vi "Hall sensor read-modify.vi"() -> ()   [LabVIEW 2013]
uses:
  <vilib>/measure/mascope.llb/Amplitude and Levels N chan.vi
  <vilib>/measure/NI_MAPro.lvlib
panel:
  in  "STOP":bool
  out "Anti-\nClockwise":bool
  out "Break\nCondition":bool
  out "Clockwise":bool
  out "No \nMagnetic\n    Field":bool
  out "North \n  Pole":bool
  out "South \n  Pole":bool
  out "PWM being applied\n(~Strength of magnetic field)":dbl
  out "Voltage Output- Hall Sensor":dynamicdata(graph)
  # "Hall Sensor Control"
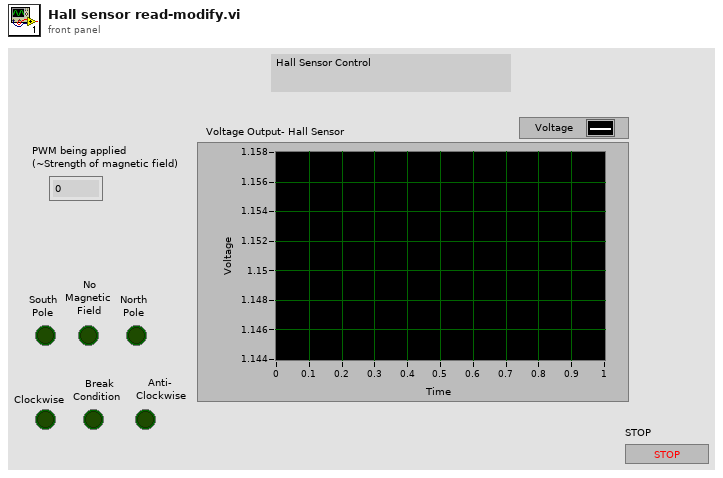
[diagram p1: front panel]
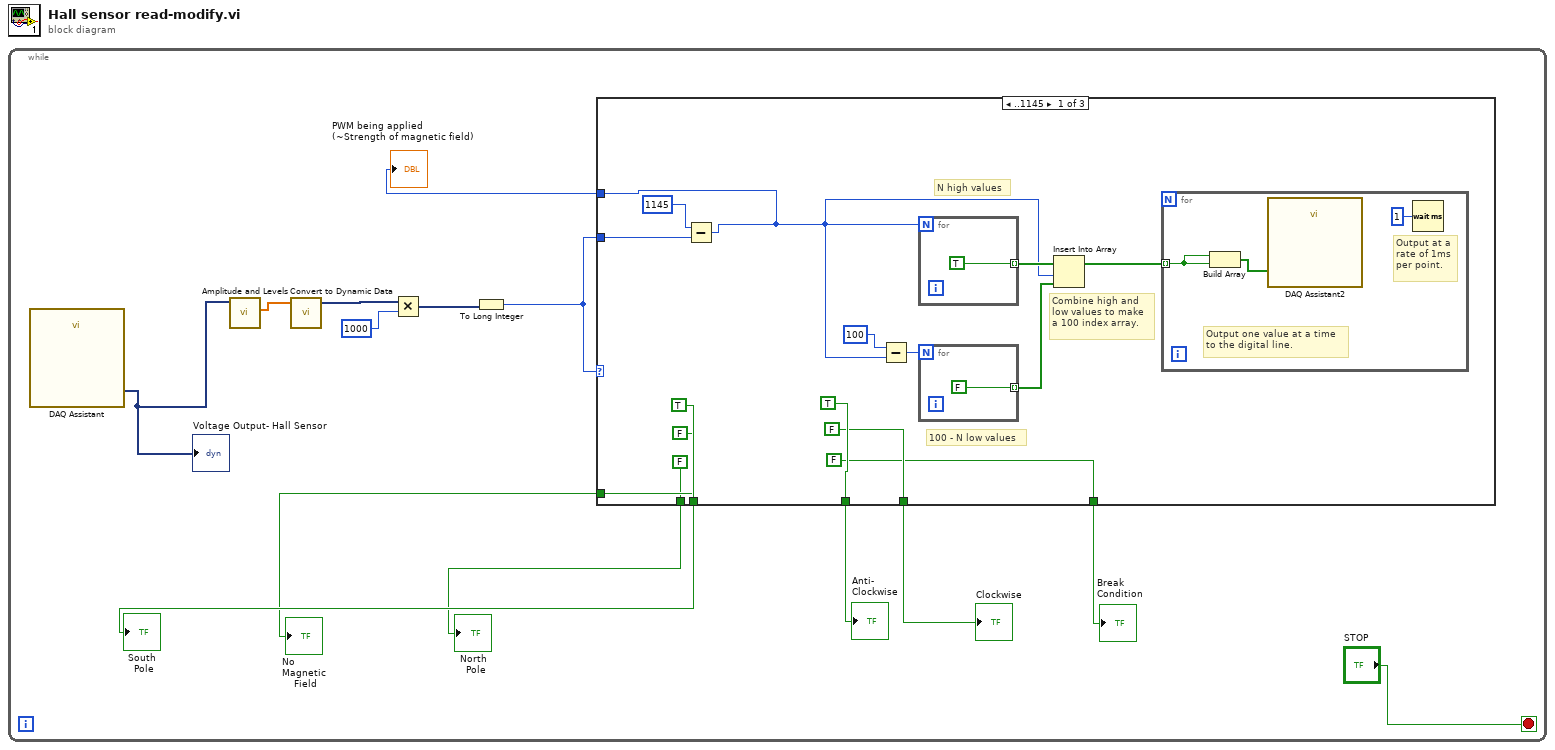
[diagram p0: block diagram]
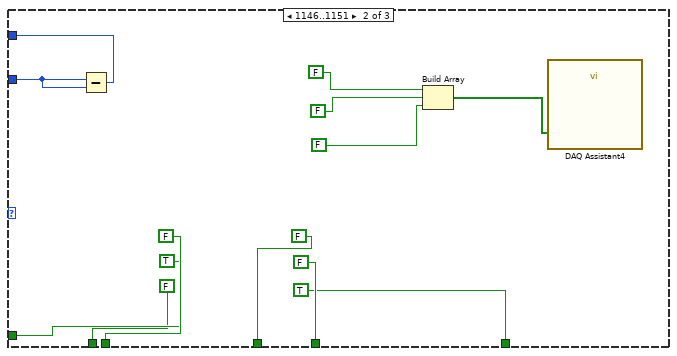
[diagram p2: hidden frame]
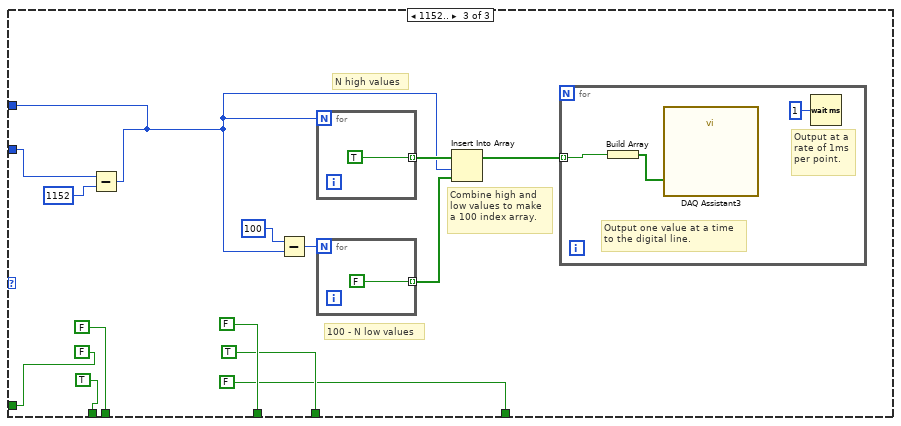
[diagram p3: hidden frame]
diagram:
  n1 = while {
    stop <- "STOP" stop-if-true
    n2 = call "DAQ Assistant"() -> ("data"=w14:dynamicdata)  [unwired: 17 in, 2 out]
    "Voltage Output- Hall Sensor" <- w14
    n3 = call-poly <vilib>:"Amplitude and Levels.vi"("signal(s) in"=w14) -> ("high state level"=w1:dbl[])  [unwired: 7 in, 3 out]
    n4 = call "Convert to Dynamic Data"("Array"=w1) -> ("Dynamic Data Type"=w12:dynamicdata)  [unwired: 3 in]
    n5 = Multiply(x=w12, y=1000) -> (x*y=w13:dynamicdata)
    n6 = To Long Integer(number=w13) -> (32bit integer=w10:i32)
    n7 = case shown="..1145" w10 {
      tunnel: w10 -> [w22 w41 w54]
      tunnel: [w21 w40 w52] -> w9
      tunnel: [TRUE FALSE FALSE] -> w8
      tunnel: [FALSE TRUE FALSE] -> w7
      tunnel: [FALSE FALSE TRUE] -> w6
      tunnel: [TRUE FALSE FALSE] -> w5
      tunnel: [FALSE FALSE TRUE] -> w4
      tunnel: [FALSE TRUE FALSE] -> w3
      frame ..1145 {
        # "Combine high and\nlow values to make\na 100 index array."
        # "100 - N low values"
        # "N high values"
        n8 = Subtract(x=1145, y=w22) -> (x-y=w21:i32)
        n9 = Subtract(x=100, y=w21) -> (x-y=w27:i32)
        n10 = for {
          N: w21 -> [_]
          tunnel: [TRUE] -> w26 mode=indexing
        }
        n11 = for {
          N: w27 -> [_]
          tunnel: [FALSE] -> w25 mode=indexing
        }
        n12 = Insert Into Array(array=w26, index=w21, new element=w25) -> (w24:bool[])
        n13 = for {
          tunnel: w24 -> [w32] mode=indexing
          # "Output at a\nrate of 1ms\nper point."
          # "Output one value at a time\nto the digital line."
          n14 = Build Array(w32, w32) -> (w31:bool[])
          n15 = call "DAQ Assistant2"("data"=w31) -> ()  [unwired: 17 in, 2 out]
          n16 = Wait (ms)(milliseconds to wait=u32 1) -> ()  [unwired: 1 out]
        }
      }
      frame 1146..1151 {
        n17 = Subtract(x=w41, y=w41) -> (x-y=w40:i32)
        n18 = Build Array(FALSE, FALSE, FALSE) -> (w42:bool[])
        n19 = call "DAQ Assistant4"("data"=w42) -> ()  [unwired: 17 in, 2 out]
      }
      frame 1152.. {
        # "Combine high and\nlow values to make\na 100 index array."
        # "100 - N low values"
        # "N high values"
        n20 = Subtract(x=w54, y=1152) -> (x-y=w52:i32)
        n21 = Subtract(x=100, y=w52) -> (x-y=w56:i32)
        n22 = for {
          N: w52 -> [_]
          tunnel: [TRUE] -> w57 mode=indexing
        }
        n23 = for {
          N: w56 -> [_]
          tunnel: [FALSE] -> w58 mode=indexing
        }
        n24 = Insert Into Array(array=w57, index=w52, new element=w58) -> (w59:bool[])
        n25 = for {
          tunnel: w59 -> [w63] mode=indexing
          # "Output at a\nrate of 1ms\nper point."
          # "Output one value at a time\nto the digital line."
          n26 = Build Array(w63) -> (w62:bool[])
          n27 = call "DAQ Assistant3"("data"=w62) -> ()  [unwired: 17 in, 2 out]
          n28 = Wait (ms)(milliseconds to wait=u32 1) -> ()  [unwired: 1 out]
        }
      }
    }
    "PWM being applied\n(~Strength of magnetic field)" <- w9
    "No \nMagnetic\n    Field" <- w7
    "South \n  Pole" <- w8
    "North \n  Pole" <- w6
    "Clockwise" <- w4
    "Break\nCondition" <- w3
    "Anti-\nClockwise" <- w5
  }
